vi "ApplyCLKdialog.vi"() -> (0 "drop?":bool, 1 "时间（分钟） 2":u32, 2 "时钟出 2":string(combo), 3 "时钟进 2":string(combo))   [LabVIEW 2015]
panel:
  in  "Cancel":bool
  in  "OK":bool
  in  "时间（分钟）":u32=90
  in  "时钟出":string(combo)="OUT1"
  in  "时钟进":string(combo)="IN1"
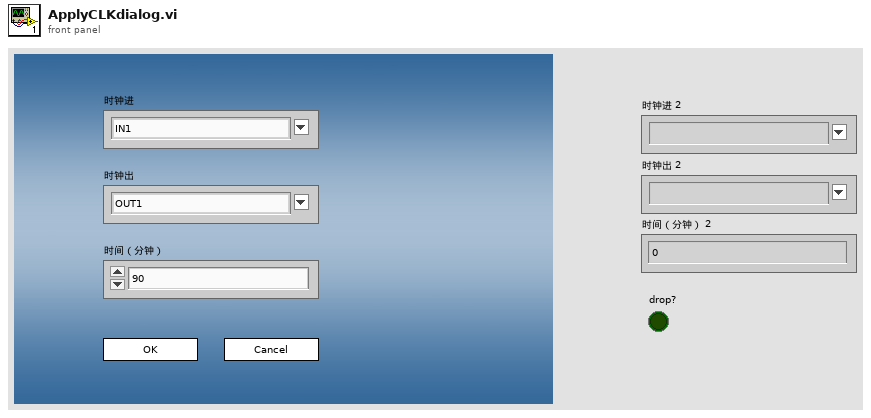
[diagram p1: front panel]
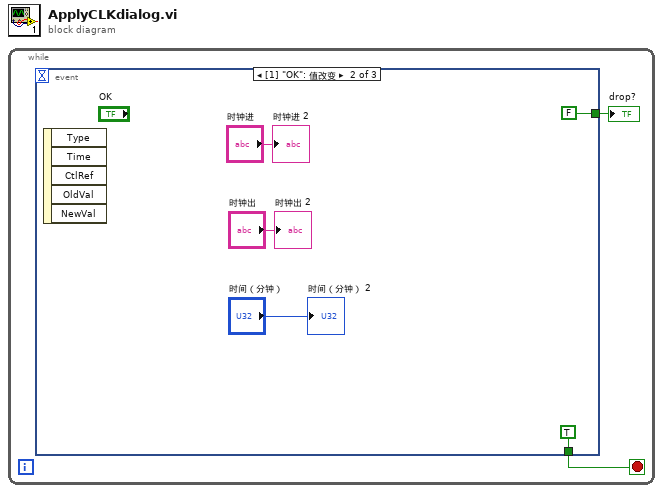
[diagram p0: block diagram]
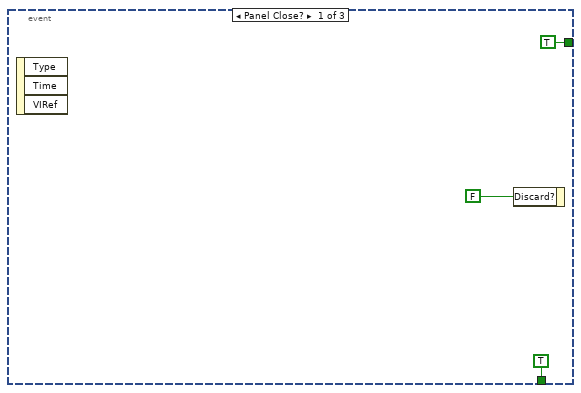
[diagram p2: hidden frame]
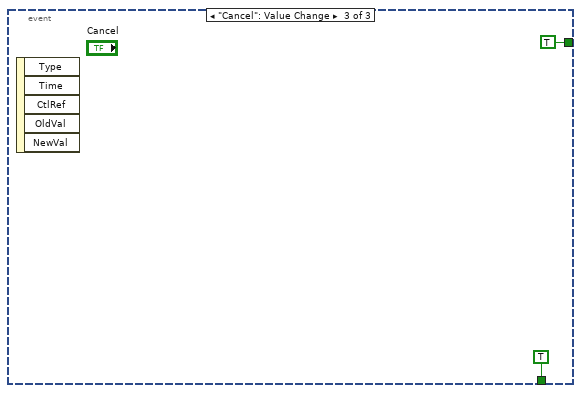
[diagram p3: hidden frame]
diagram:
  n1 = while {
    stop <- w1 stop-if-true
    n2 = event shown="[1] \"OK\": 值改变" {
      selector: _ -> [_ _ _]
      dyn-events: _ -> [_ _ _]
      timeout: _ -> [_ _ _]
      tunnel: [TRUE FALSE TRUE] -> w2
      tunnel: [TRUE TRUE TRUE] -> w1
      event Panel Close? {
        n3 = event-data() -> ()  [unwired: 1 in, 3 out]
        n4 = event-data("Discard?"=FALSE ("放弃？")) -> ()  [unwired: 1 in, 1 out]
      }
      event "OK": Value Change {
        n5 = event-data() -> ()  [unwired: 1 in, 5 out]
        "时钟进 2" <- "时钟进"
        "时钟出 2" <- "时钟出"
        "时间（分钟） 2" <- "时间（分钟）"
      }
      event "Cancel": Value Change {
        n6 = event-data() -> ()  [unwired: 1 in, 5 out]
      }
    }
    "drop?" <- w2
  }
